vi "string_time_to_integer.vi"(8 "error in (no error)":errorcluster, 10 "Time string (mm:ss)":string) -> (0 "error out":errorcluster, 2 "Time (s)":u16)   [LabVIEW 2018]
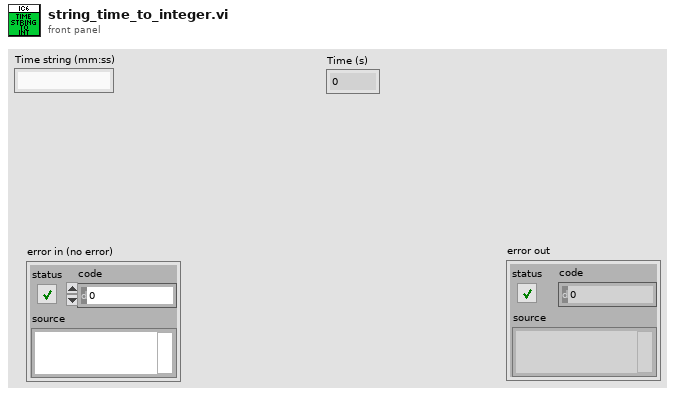
[diagram p1: front panel]
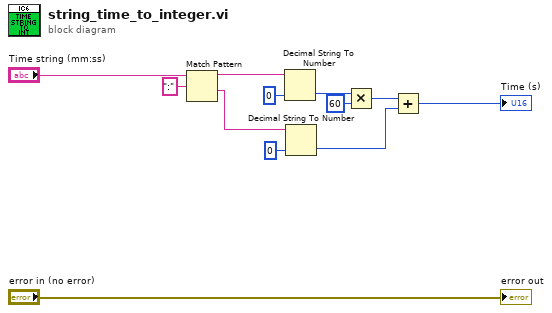
[diagram p0: block diagram]
diagram:
  n1 = Match Pattern(string="Time string (mm:ss)", regular expression=":") -> (before substring=w9:string, after substring=w3:string)  [unwired: 1 in, 2 out]
  n2 = Decimal String To Number(string=w9, default (0L)=u16 0 ("default (0 I32)")) -> (number=w7:u16)  [unwired: 1 in, 1 out]
  n3 = Decimal String To Number(string=w3, default (0L)=u16 0 ("default (0 I32)")) -> (number=w2:u16)  [unwired: 1 in, 1 out]
  n4 = Multiply(x=w7, y=u16 60) -> (x*y=w5:u16)
  n5 = Add(x=w5, y=w2) -> (x+y=→"Time (s)":u16)
  "error out" <- "error in (no error)"
